vi "Close.vi"(8 "error in (no error)":errorcluster, 11 "MKS MW in":refnum<class "PL MKS MW.lvclass">) -> (0 "error out":errorcluster)   [LabVIEW 2015, in "PL MKS MW.lvclass"]
doc: "Closes connection to device."
uses:
  PL MKS MW.lvclass
  PL MKS MW.lvclass/PL MKS MW.ctl
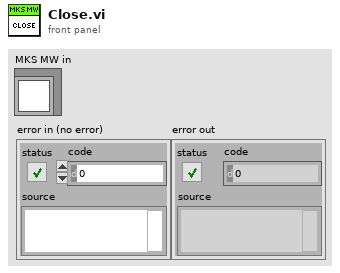
[diagram p1: front panel]
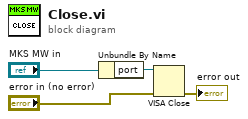
[diagram p0: block diagram]
diagram:
  n1 = Unbundle By Name("MKS MW in") -> ("port"=w3:refnum<visa-resource-name>)
  n2 = VISA Close(VISA resource name=w3, error in (no error)="error in (no error)") -> (error out=→"error out":errorcluster)
